vi "LED_W.vi"(2 "error INPUT":errorcluster, 3 "VISA resource Input":refnum<visa-resource-name>, 4 "Option  Led color":dbl=1.0 min=1.0 max=3.0) -> (0 "error out":errorcluster, 1 "VISA resource name out":refnum<visa-resource-name>)   [LabVIEW 2011]
panel:
  out "unsigned byte array":u8[](array[numeric])
  out "x+y":dbl
  out "Read LED command":u8[](array[numeric])
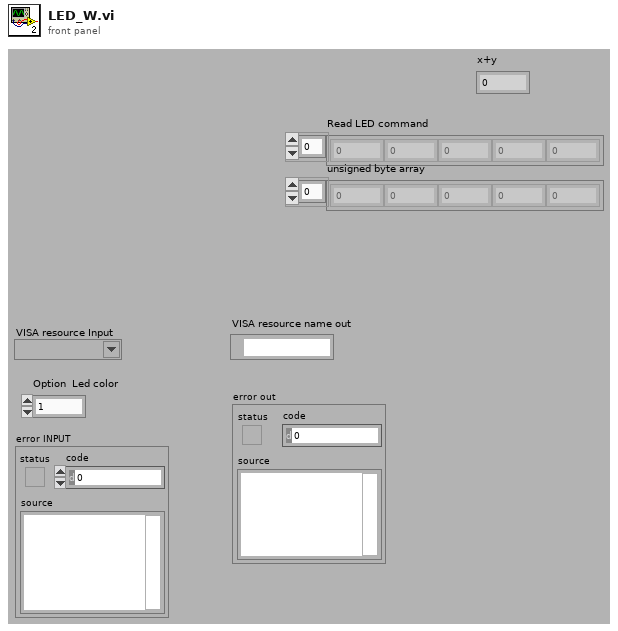
[diagram p1: front panel]
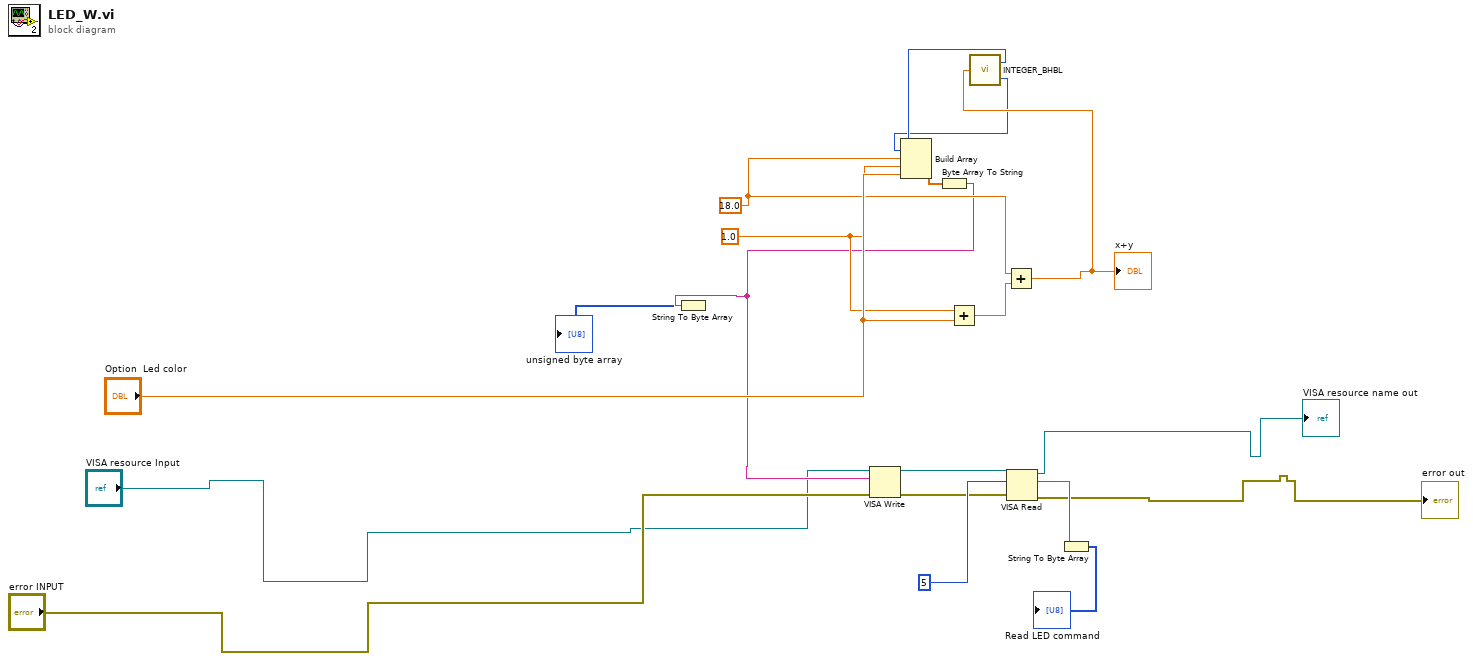
[diagram p0: block diagram]
diagram:
  w11 = 1.0 ("element")
  w9 = 18.0 ("element")
  n1 = Add(x=w11, y="Option  Led color") -> (x+y=w10:dbl)
  n2 = Add(x=w9, y=w10) -> (x+y=w8:dbl)
  "x+y" <- w8
  n3 = call "INTEGER_BHBL.vi"("int16"=w8) -> ("Lvalue"=w6:u8, "HValue"=w7:u8)
  n4 = Build Array(w7, w6, w9, w11, "Option  Led color") -> (w13:dbl[])
  n5 = Byte Array To String(unsigned byte array=w13) -> (string=w5:string)
  n6 = String To Byte Array(string=w5) -> (unsigned byte array=→"unsigned byte array":u8[])
  n7 = VISA Write(VISA resource name="VISA resource Input", write buffer=w5, error in (no error)="error INPUT") -> (VISA resource name out=w14:refnum<visa-resource-name>, error out=w15:errorcluster)  [unwired: 1 out]
  n8 = VISA Read(VISA resource name=w14, byte count=u32 5, error in (no error)=w15) -> (VISA resource name out=→"VISA resource name out":refnum<visa-resource-name>, read buffer=w17:string, error out=→"error out":errorcluster)  [unwired: 1 out]
  n9 = String To Byte Array(string=w17) -> (unsigned byte array=→"Read LED command":u8[])
